vi "Recursive Child Symbol Reader.vi"(8 "error in (no error)":errorcluster, 9 ".NET TcAdsSymbolInfo":refnum<k24>, 11 "TwinCAT ADS in":refnum<class "TwinCAT ADS.lvclass">) -> (0 "error out":errorcluster, 1 "Symbols Information":T1[](array[typedef]) {"Type ID" items=["ADST_VOID"=0, "ADST_INT16"=2, "ADST_INT32"=3, "ADST_REAL32"=4, "ADST_REAL64"=5, "ADST_INT8"=16, "ADST_UINT8"=17, "ADST_UINT16"=18, "ADST_UINT32"=19, "ADST_INT64"=20, "ADST_UINT64"=21, "ADST_STRING"=30, "ADST_WSTRING"=31, "ADST_REAL80"=32, "ADST_BIT"=33, "ADST_MAXTYPES"=34, "ADST_BIGTYPE"=65]; "Type Category" items=["Unknown, None"=0, "Primitive"=1, "Alias"=2, "Enum"=3, "Array"=4, "Struct"=5, "FunctionBlock"=6, "Program"=7, "Function"=8, "SubRange"=9, "String"=10, "Bitset"=12, "Pointer"=13, "Union"=14, "Reference"=15, "Interface"=16]}, 3 "TwinCAT ADS out":refnum<class "TwinCAT ADS.lvclass">)   [LabVIEW 2018, in "TwinCAT ADS.lvclass"]
uses:
  TwinCAT ADS.lvclass
  TwinCAT.Ads
  Controls/Symbol Information.ctl
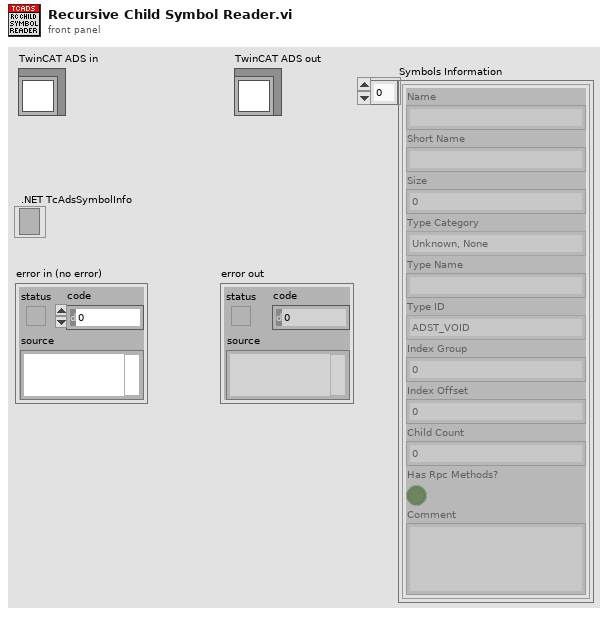
[diagram p1: front panel]
types:
  T1 = typedef "TwinCAT ADS.lvclass/Symbol Information.ctl" = cluster{"Name":string, "Short Name":string, "Size":i32, "Type Category":i32, "Type Name":string, "Type ID":i32, "Index Group":i64, "Index Offset":i64, "Child Count":i32, "Has Rpc Methods?":bool, "Comment":string}
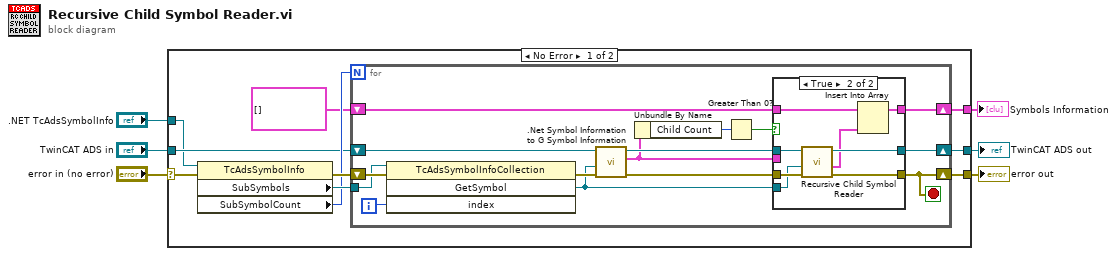
[diagram p0: block diagram]
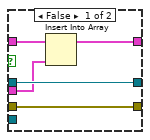
[diagram p2: hidden frame]
diagram:
  n1 = case shown="No Error" "error in (no error)" {
    selector: "error in (no error)" -> [w12 w46]
    tunnel: [w9 w46] -> w5
    tunnel: [w10 w45] -> w3
    tunnel: "TwinCAT ADS in" -> [w13 w45]
    tunnel: ".NET TcAdsSymbolInfo" -> [w11 _]
    tunnel: [w7 _] -> w1
    frame No Error {
      n2 = property class="TcAdsSymbolInfo"(reference=w11, error in=w12) -> (error out=w16:errorcluster, "SubSymbols"=w15:refnum<k24>, "SubSymbolCount"=w14:i32)  [unwired: 1 out]
      n3 = for {
        N: w14 -> [_]
        tunnel: w15 -> [w30]
        shift-right: [w17] -> w9
        shift-left: w16 -> [w31]
        shift-right: [w18] -> w7
        shift-left: T1[] [] -> [w19]
        shift-right: [w20] -> w10
        shift-left: w13 -> [w27]
        i -> [w29]
        stop <- w17 stop-if-true
        n4 = invoke class="TcAdsSymbolInfoCollection" method="GetSymbol"(reference=w30, error in=w31, "index"=w29) -> (error out=w28:errorcluster, "GetSymbol"=w22:refnum<k24>)  [unwired: 1 in, 2 out]
        n5 = call ".Net Symbol Information to G Symbol Information.vi"("TwinCAT ADS in"=w27, ".NET ITcAdsSymbolInfo refnum"=w22, "error in (no error)"=w28) -> ("TwinCAT ADS out"=w24:refnum<class "TwinCAT ADS.lvclass">, "Symbol Information"=w21:T1, "error out"=w23:errorcluster)  [unwired: 5 in]
        n6 = Unbundle By Name(w21) -> ("Child Count"=w26:i32)
        n7 = Greater Than 0?(x=w26) -> (x > 0?=w25:bool)
        n8 = case shown="True" w25 {
          tunnel: w24 -> [w36 w43]
          tunnel: w23 -> [w35 w44]
          tunnel: w22 -> [_ w38]
          tunnel: w21 -> [w32 _]
          tunnel: [w36 w41] -> w20
          tunnel: [w35 w42] -> w17
          tunnel: w19 -> [w34 w40]
          tunnel: [w33 w39] -> w18
          frame False {
            n9 = Insert Into Array(array=w34, new element=w32) -> (w33:T1[])  [unwired: 1 in]
          }
          frame True {
            n10 = call "Recursive Child Symbol Reader.vi"("error in (no error)"=w44, ".NET TcAdsSymbolInfo"=w38, "TwinCAT ADS in"=w43) -> ("error out"=w42:errorcluster, "Symbols Information"=w37:T1[], "TwinCAT ADS out"=w41:refnum<class "TwinCAT ADS.lvclass">)  [unwired: 6 in]
            n11 = Insert Into Array(array=w40, new element=w37) -> (w39:T1[])  [unwired: 1 in]
          }
        }
      }
    }
    frame Error {
    }
  }
  "error out" <- w5
  "TwinCAT ADS out" <- w3
  "Symbols Information" <- w1
